vi "Monochromator.vi"() -> ()   [LabVIEW 2018]
uses:
  classes/Tushars Events Toolkit/Software/Modules/EventClient_ObjectReference.ctl
  Controls/Data highway.ctl
  Controls/LED intensity Command.ctl
  Strict Type Controls/Settings Operation.ctl
  Controls/API Command.ctl
  42e5cc38-9382-4005-a5db-d423bf5d2c61.vi
  dcdd8a02-0f9a-4db7-9287-66503d747d34.vi
  classes/Variable Manager/VariableManager_Bool.vi
  Controls/Support Global.vi
  classes/Variable Manager/VariableManager_I32.vi
  classes/Variable Manager/VariableManager_Double.vi
panel:
  out "Quit":bool
  out "error out":errorcluster
  in  "error in (no error)":errorcluster
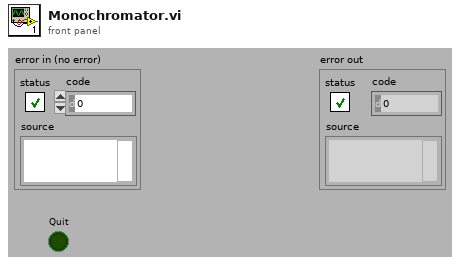
[diagram p1: front panel]
types:
  T1 = typedef "Data highway.ctl" = cluster{"MonoCr Port":refnum<visa-resource-name>, "Grating Selection":enum16{"Grating@1", "Grating@2"}, "Connection?":bool, "LED Comm":T2, "Intensity Value":i32, "Grating Number":i32, "Wavenumber":i32, "Slit Width":i32, "Filter Num":i32, "Grating Density":i32, "Wavelength(nm)":i32, "offset":dbl}
  T2 = typedef "LED intensity Command.ctl" = enum16{"LED@1", "LED@2"}
  T3 = typedef "EventClient_ObjectReference.ctl" = refnum<k1>
  T4 = typedef "API Command.ctl" = enum16{"Init", "Device Check", "Grating Density@1", "Grating Density@2", "SetWavelength", "Filter Selection", "Shutter open", "Shutter close", "LED Intensity", "Set Grating", "Slit Width", "Stop running", "Reset Mono", "Close"}
  T5 = typedef "Settings Operation.ctl" = enum8{"Get Value", "Set Value", "Read File", "Write File", "Write Stored Value"}
  T6 = typedef "Settings.ctl" = cluster{"Mono Cr":cluster{"Port":refnum<visa-resource-name>, "baud rate":u32, "data bits":u16, "parity":enum16{"None", "Odd", "Even", "Mark", "Space"}, "stop bits":u16, "flow control":u16, "timeout":u32}, "Merlin":cluster{"Port":refnum<visa-resource-name>, "baud rate":u32, "data bits":u16, "parity":enum16{"None", "Odd", "Even", "Mark", "Space"}, "stop bits":u16, "flow control":u16, "timeout":u32}}
  T7 = typedef "Wavelength Cluster Variable.ctl" = cluster{"Filter Num":i32, "Grating Density":i32, "Wavelength(nm)":i32}
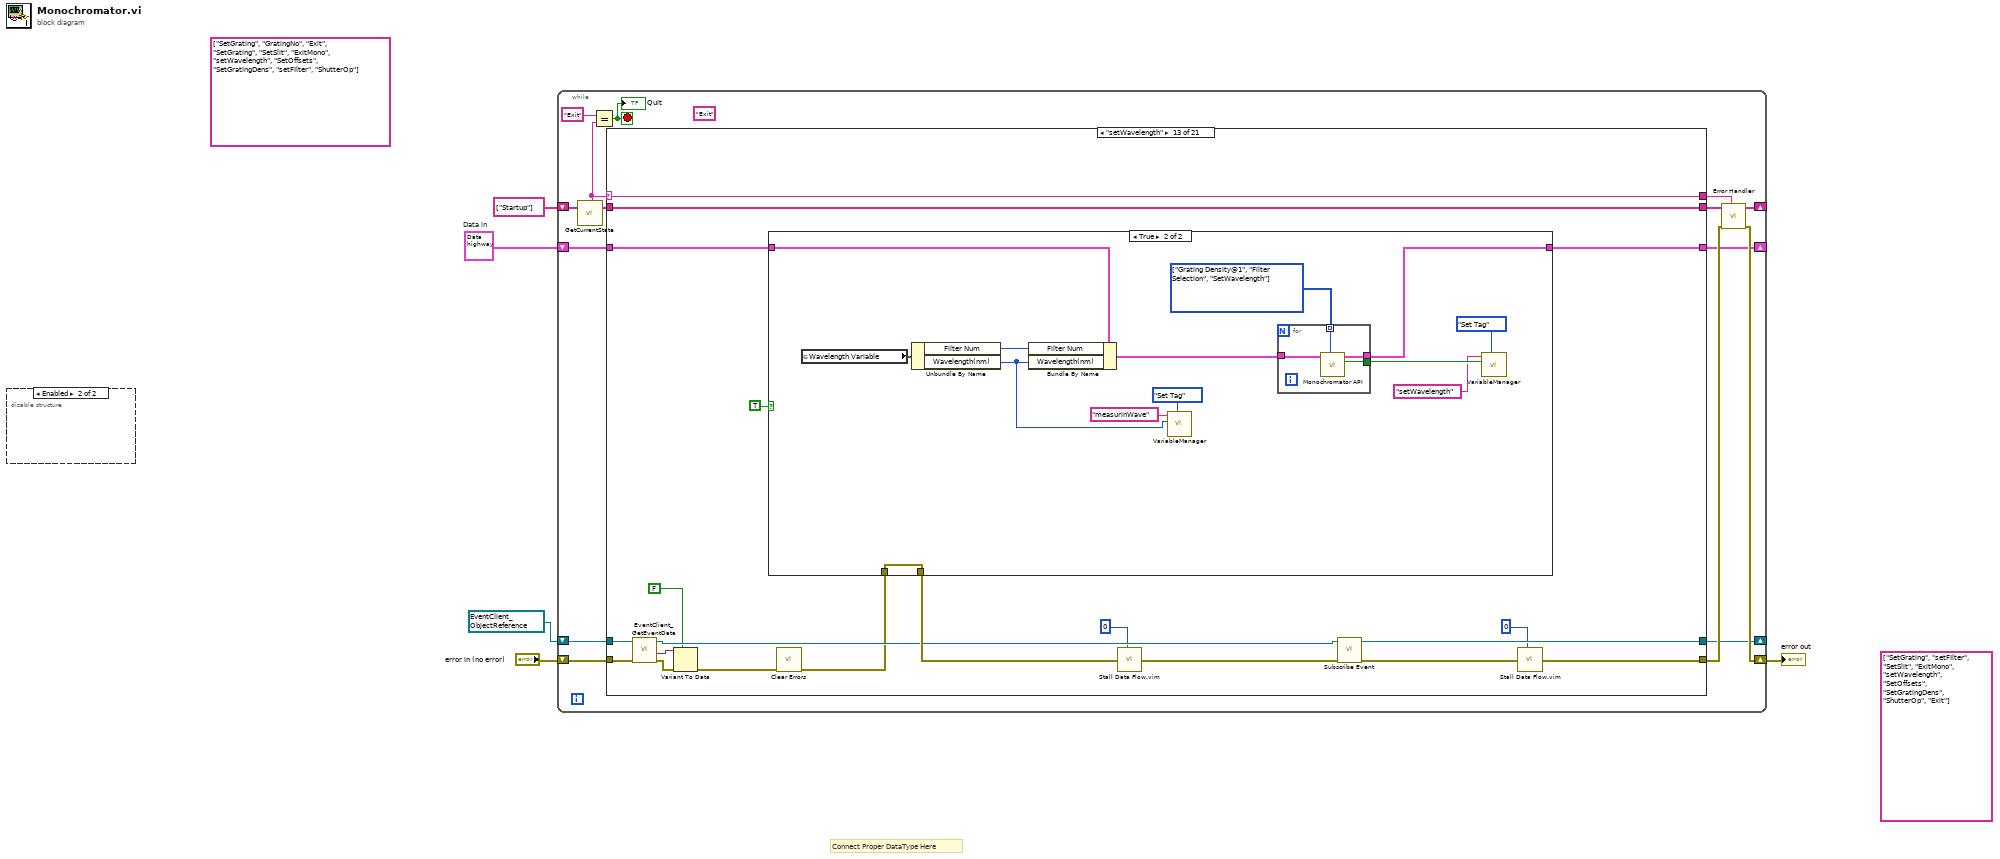
[diagram p0: block diagram]
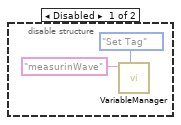
[diagram p2: hidden frame]
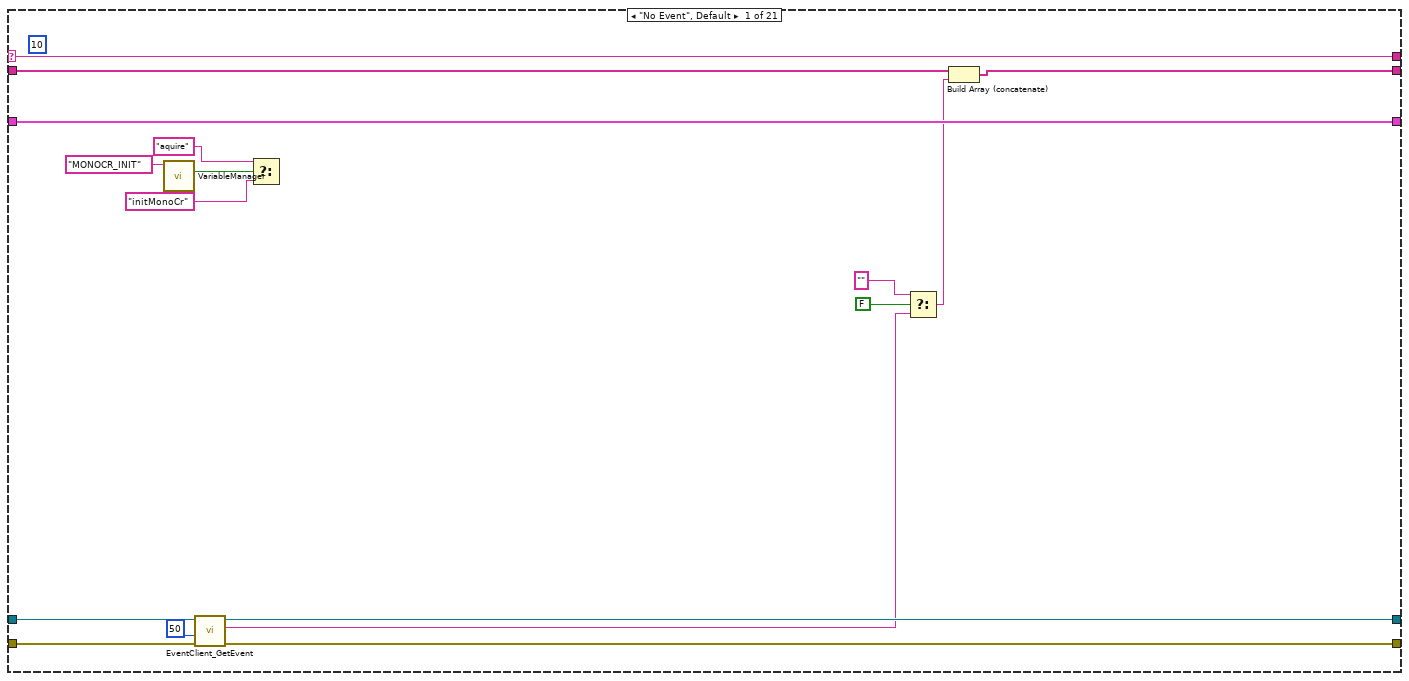
[diagram p3: hidden frame]
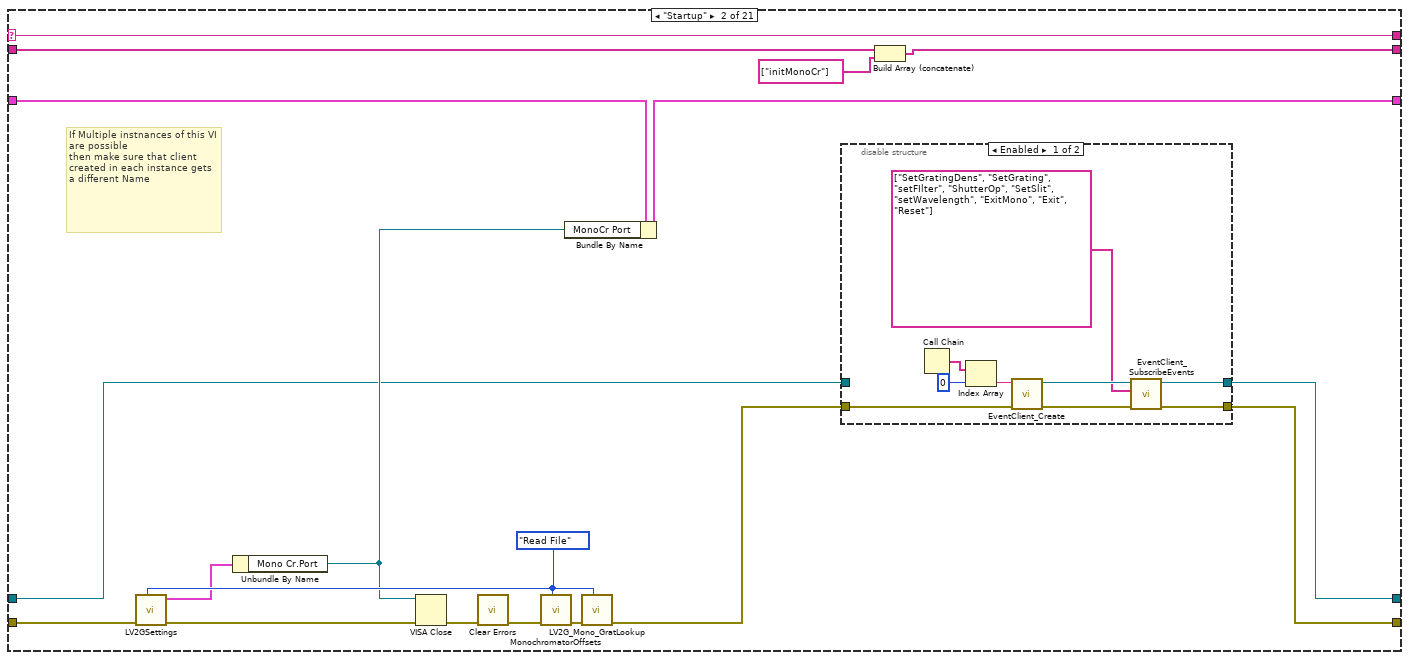
[diagram p4: hidden frame]
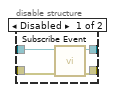
[diagram p6: hidden frame]
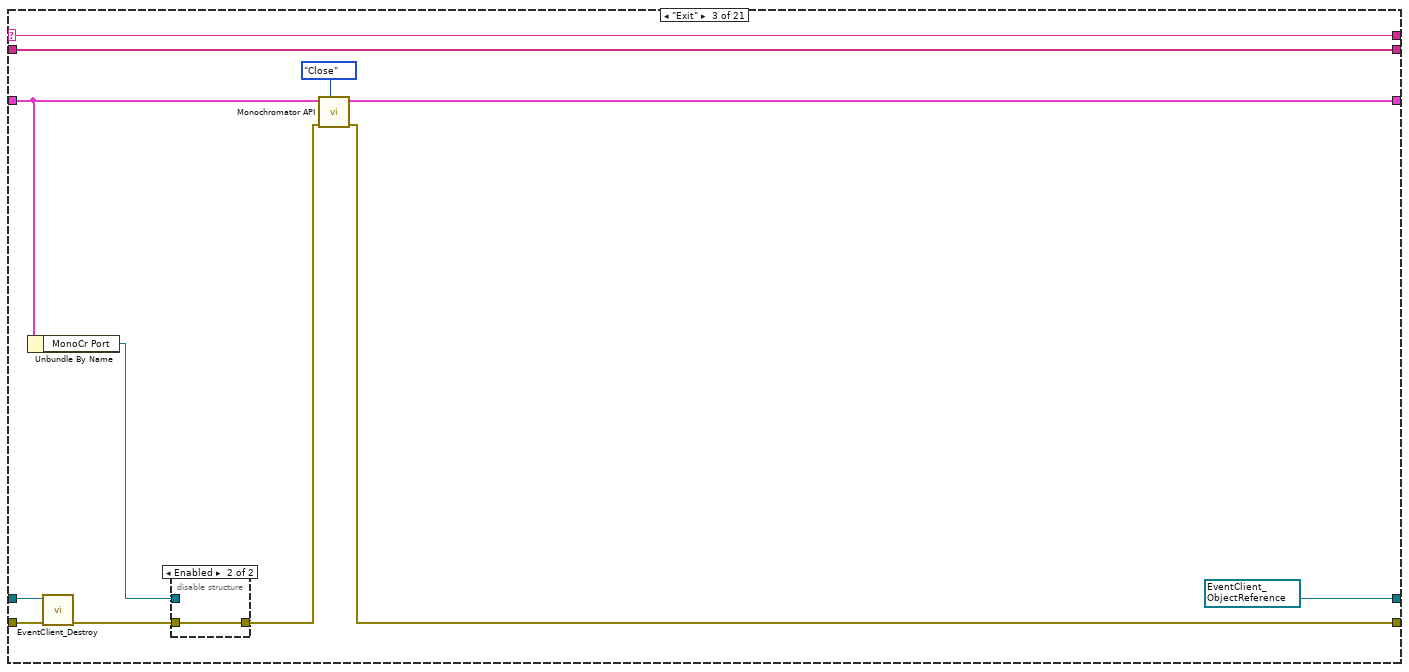
[diagram p7: hidden frame]
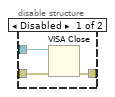
[diagram p8: hidden frame]
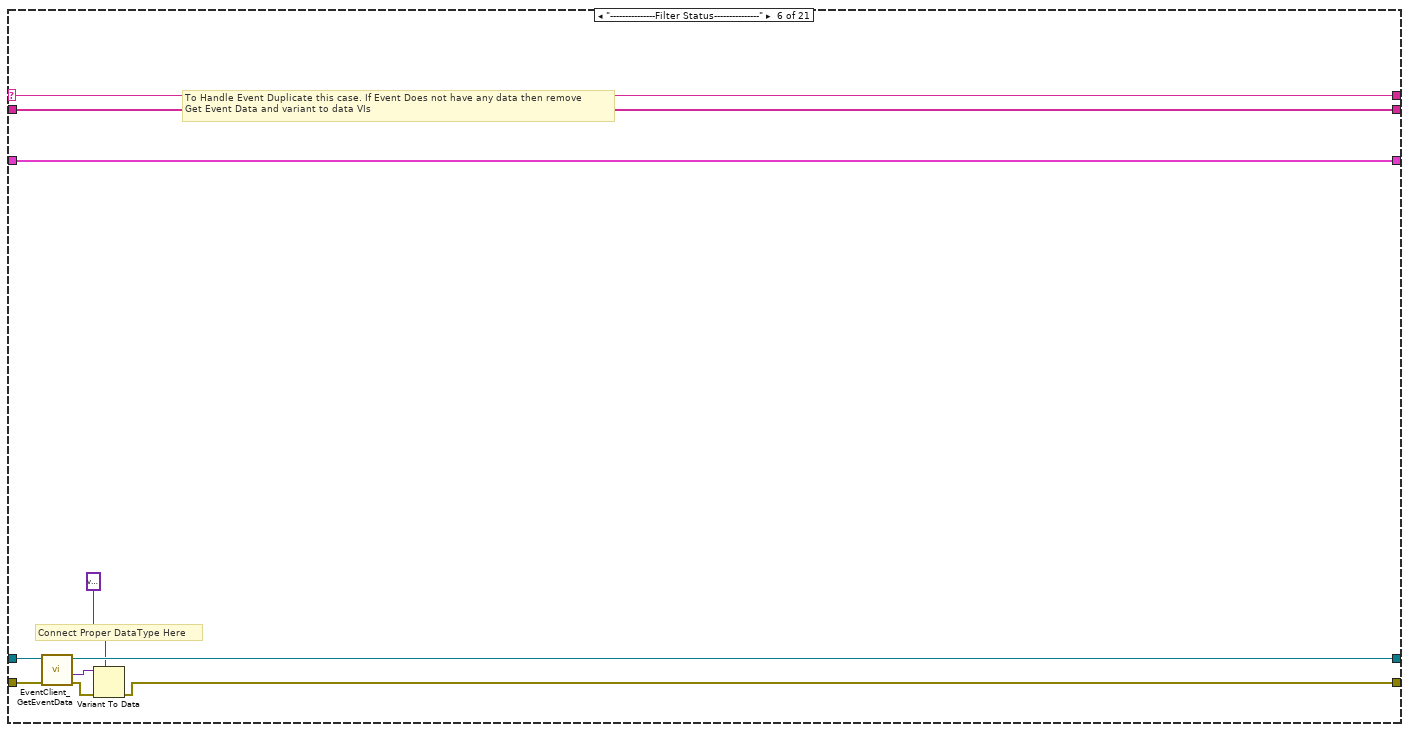
[diagram p11: hidden frame]
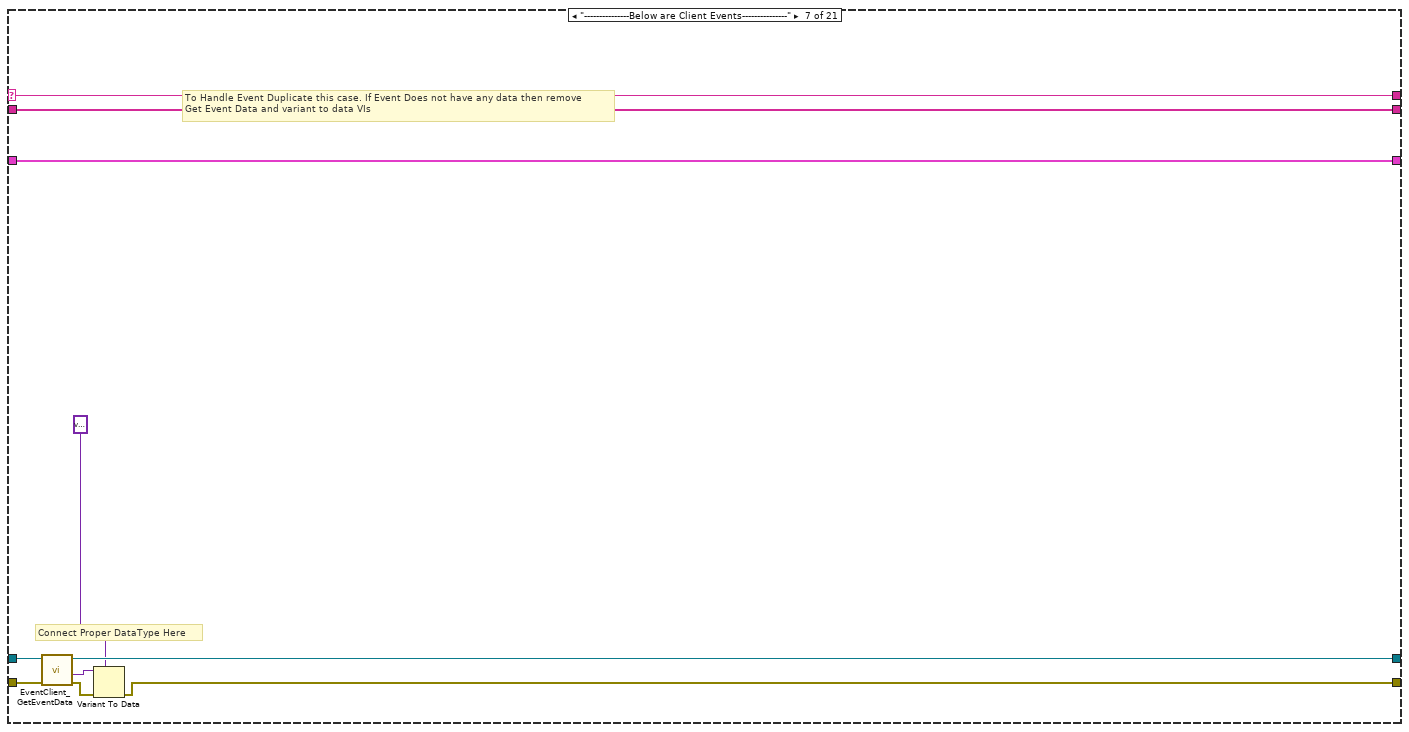
[diagram p12: hidden frame]
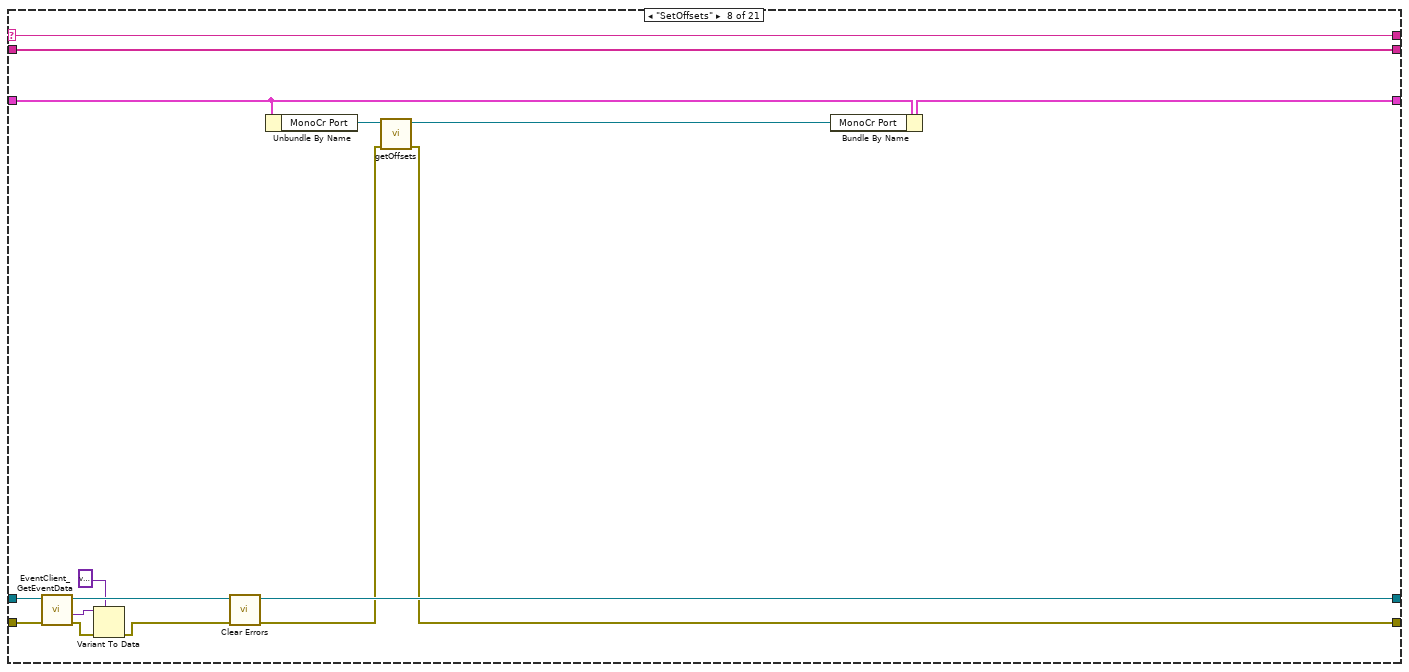
[diagram p13: hidden frame]
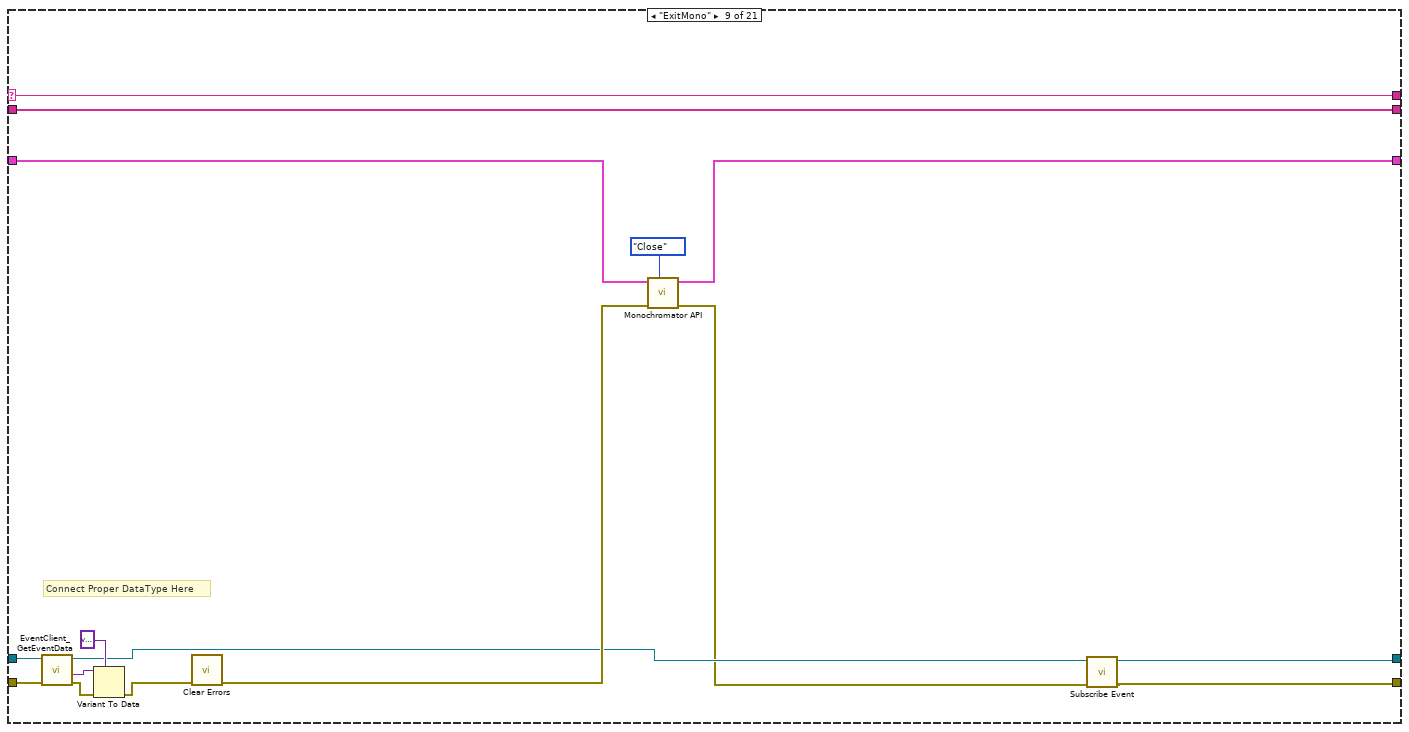
[diagram p14: hidden frame]
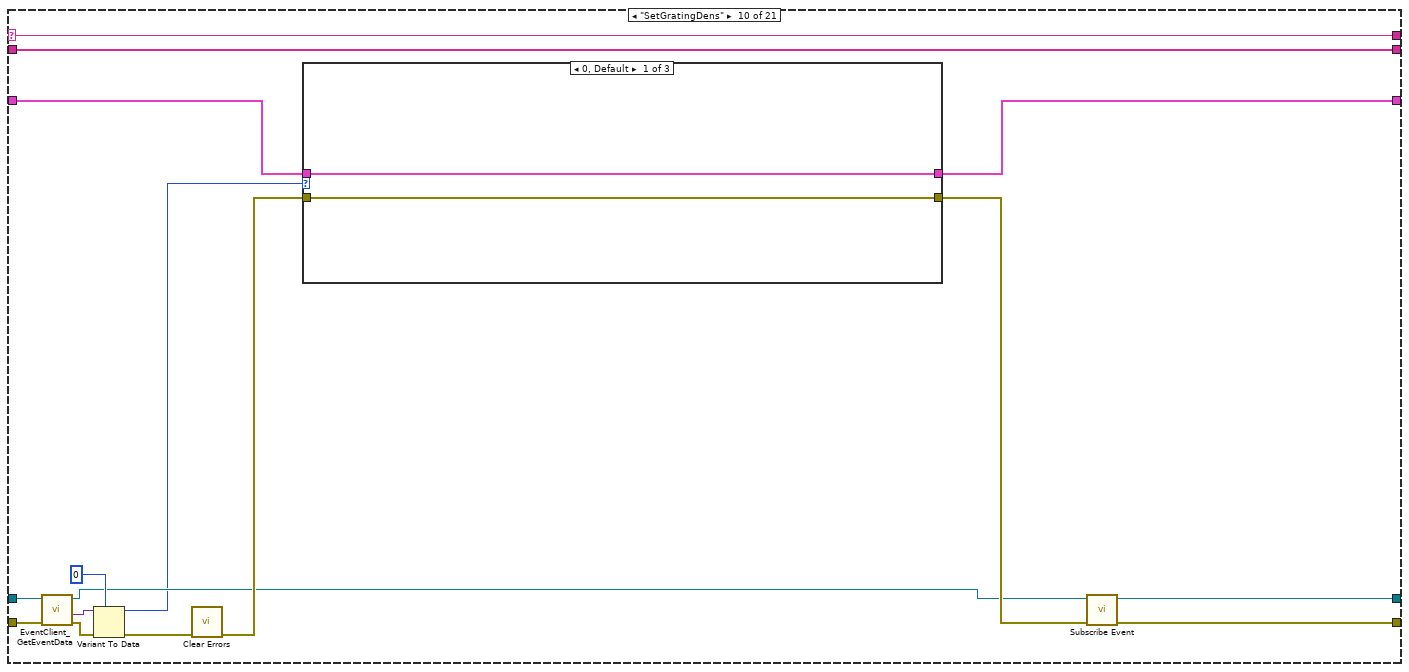
[diagram p15: hidden frame]
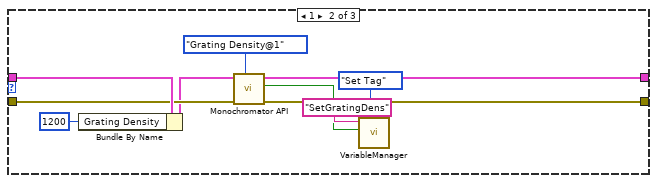
[diagram p16: hidden frame]
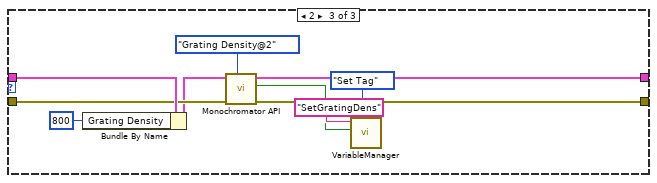
[diagram p17: hidden frame]
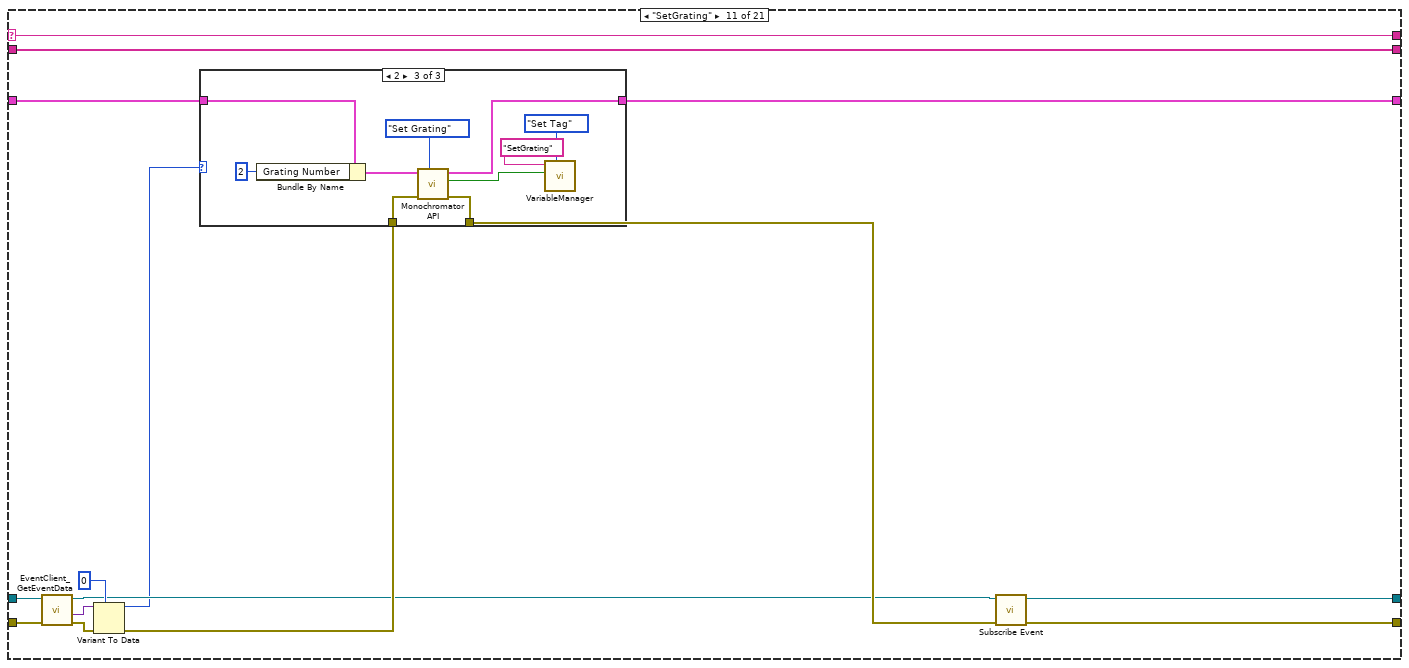
[diagram p18: hidden frame]
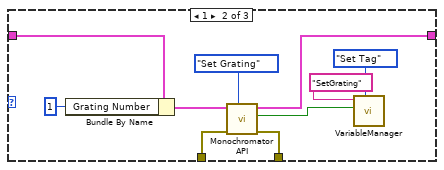
[diagram p20: hidden frame]
diagram:
  w1 = T1 {"MonoCr Port"="COM3", "Grating Selection"=enum."Grating@1", "Connection?"=TRUE, "LED Comm"=enum."LED@1", "Intensity Value"=20, "Grating Number"=1, "Wavenumber"=0, "Slit Width"=8, "Filter Num"=3, "Grating Density"=1200, "Wavelength(nm)"=532, "offset"=0.0}  # Data in
  (unwired) string[] ["SetGrating", "GratingNo", "Exit", "SetGrating", "SetSlit", "ExitMono", "setWavelength", "SetOffsets", "SetGratingDens", "setFIlter", "ShutterOp"] ("Events")
  (unwired) string[] ["SetGrating", "setFIlter", "SetSlit", "ExitMono", "setWavelength", "SetOffsets", "SetGratingDens", "ShutterOp", "Exit"] ("Events")
  w2 = T3 refnum items=["EventClient"] ("reference")
  # "Connect Proper DataType Here"
  n1 = disable-structure shown="Enabled" {
    frame Disabled {
      n2 = call-poly "VariableManager.vi"("Operation"=enum16{"Get Tag", "Set Tag"}."Set Tag", "Tag"="measurinWave") -> ()  [unwired: 5 in, 5 out]
    }
    frame Enabled {
    }
  }
  n3 = while {
    shift-right: [w18] -> _
    shift-left: string[] ["Startup"] ("State Array Out") -> [w22]
    shift-right: [w14] -> w3
    shift-left: "error in (no error)" -> [w15]
    shift-right: [w11] -> _
    shift-left: w2 -> [w10]
    shift-right: [w8] -> _
    shift-left: w1 -> [w9]
    stop <- w19 stop-if-true
    (unwired) "Exit" ("x")
    n4 = call "GetCurrentState.vi"("State Array In"=w22) -> ("Current State"=w12:string, "State Array Out"=w21:string[])  [unwired: 17 in]
    n5 = Equal?(x="Exit", y=w12) -> (x = y?=w19:bool)
    "Quit" <- w19
    n6 = case shown="\"setWavelength\"" w12 {
      selector: w12 -> [w39 w57 w88 w96 w101 w111 w121 w136 w152 w168 w205 w242 w344 w378 w450 w468 w483 w488 w507 w512 w530]
      tunnel: w21 -> [w31 w56 w87 w97 w102 w112 w122 w137 w153 w169 w206 w243 w345 w379 w451 w469 w484 w489 w502 w511 w517]
      tunnel: [w34 w55 w87 w97 w102 w112 w122 w137 w153 w169 w206 w243 w345 w379 w451 w469 w484 w489 w502 w511 w514] -> w17
      tunnel: [w36 w53 w78 w95 w100 w107 w117 w123 w139 w157 w195 w232 w329 w367 w435 w459 w482 w485 w501 w510 errorcluster {"status"=FALSE, "code"=0, "source"=""} ("error in (no error)")] -> w13
      tunnel: [w39 w57 w88 w96 w101 w111 w121 w136 w152 w168 w205 w242 w344 w378 w450 w468 w483 w488 w507 w512 w530] -> w16
      tunnel: w15 -> [w37 w50 w85 w95 w100 w109 w119 w134 w150 w166 w203 w240 w342 w376 w448 w466 w482 w485 w503 w510 w518]
      tunnel: [w35 w52 w84 w94 w99 w105 w115 w131 w138 w156 w194 w231 w334 w368 w434 w458 w481 w487 w506 w509 w516] -> w11
      tunnel: w10 -> [w38 w41 w86 w94 w99 w110 w120 w135 w151 w167 w204 w241 w343 w377 w449 w467 w481 w487 w506 w509 w516]
      tunnel: w9 -> [w32 w51 w80 w93 w98 w103 w113 w127 w144 w160 w200 w237 w339 w373 w445 w463 w480 w486 w500 w508 w515]
      tunnel: [w32 w46 w77 w93 w98 w103 w113 w126 w143 w162 w199 w236 w338 w372 w444 w462 w480 w486 w499 w508 w515] -> w8
      frame "No Event", Default {
        (unwired) 10
        n7 = call-poly "VariableManager.vi"("Tag"="MONOCR_INIT") -> ("Value out"=w28:bool)  [unwired: 7 in, 3 out]
        n8 = call "EventClient_GetEvent.vi"("error in (no error)"=w37, "timeout in ms (-1)"=50, "reference"=w38) -> ("error out"=w36:errorcluster, "Name"=w30:string, "reference out"=w35:T3)  [unwired: 4 in, 2 out]
        n9 = Select(t="aquire" ("Tag"), s=w28, f="initMonoCr" ("Tag")) -> ()  [unwired: 1 out]
        n10 = Select(t="", s=FALSE, f=w30) -> (s? t:f=w29:string)
        n11 = Build Array (concatenate)(w31, w29) -> (w34:string[])
      }
      frame "Startup" {
        w49 = Settings_Operation."Read File" ("Operation")
        # "If Multiple instnances of this VI are possible \nthen make sure that client created in each instance gets a different Name"
        n12 = call "LV2GSettings.vi"("Operation"=w49, "error in (no error)"=w50) -> ("error out"=w45:errorcluster, "Settings out"=w40:T6)  [unwired: 8 in]
        n13 = Unbundle By Name(w40) -> ("Mono Cr.Port"=w43:refnum<visa-resource-name>)
        n14 = VISA Close(VISA resource name=w43, error in (no error)=w45) -> (error out=w44:errorcluster)
        n15 = call <vilib>:"Clear Errors.vi"("error in (no error)"=w44) -> ("error out"=w42:errorcluster)  [unwired: 5 in, 1 out]
        n16 = call "MonochromatorOffsets.vi"("Operation"=w49, "error in (no error)"=w42) -> ("error out"=w48:errorcluster)  [unwired: 6 in, 3 out]
        n17 = Bundle By Name(cluster=w51, "MonoCr Port"=w43) -> (w46:T1)
        n18 = call "LV2G_Mono_GratLookup.vi"("Operation"=w49, "error in (no error)"=w48) -> ("error out"=w47:errorcluster)  [unwired: 7 in, 2 out]
        n19 = disable-structure shown="Enabled" {
          disable-tunnel: [w62 w68] -> w53
          disable-tunnel: [w60 w69] -> w52
          disable-tunnel: w47 -> [w59 w70]
          disable-tunnel: w41 -> [_ w67]
          frame Enabled {
            n20 = Call Chain() -> (call chain=w66:string[])
            n21 = Index Array(array=w66, index=0) -> (element=w64:string)
            n22 = call "EventClient_Create.vi"("error in (no error)"=w59, "Instance Name"=w64) -> ("error out"=w63:errorcluster, "reference"=w61:T3)  [unwired: 8 in]
            n23 = call "EventClient_SubscribeEvents.vi"("error in (no error)"=w63, "Events"=string[] ["SetGratingDens", "SetGrating", "setFIlter", "ShutterOp", "SetSlit", "setWavelength", "ExitMono", "Exit", "Reset"], "reference"=w61) -> ("error out"=w62:errorcluster, "reference out"=w60:T3)  [unwired: 7 in]
          }
          frame Disabled {
            n24 = disable-structure shown="Enabled" {
              disable-tunnel: w70 -> [w74 w75]
              disable-tunnel: [w73 w76] -> w69
              disable-tunnel: [w72 w75] -> w68
              disable-tunnel: w67 -> [w71 w76]
              frame Disabled {
                n25 = call "Subscribe Event.vi"("error in (no error)"=w74, "reference in"=w71) -> ("error out"=w72:errorcluster, "reference out"=w73:T3)  [unwired: 8 in]
              }
              frame Enabled {
              }
            }
          }
        }
        n26 = Build Array (concatenate)(w56, string[] ["initMonoCr"] ("State Array Out")) -> (w55:string[])
      }
      frame "Exit" {
        w84 = T3 refnum items=["EventClient"] ("reference out")
        n27 = Unbundle By Name(w80) -> ("MonoCr Port"=w82:refnum<visa-resource-name>)
        n28 = call "EventClient_Destroy.vi"("error in (no error)"=w85, "reference"=w86) -> ("error out"=w83:errorcluster)  [unwired: 9 in]
        n29 = disable-structure shown="Enabled" {
          disable-tunnel: w83 -> [w91 w92]
          disable-tunnel: w82 -> [w90 _]
          disable-tunnel: [w89 w92] -> w79
          frame Disabled {
            n30 = VISA Close(VISA resource name=w90, error in (no error)=w91) -> (error out=w89:errorcluster)
          }
          frame Enabled {
          }
        }
        n31 = call "Monochromator API.vi"("Comm"=API_Command."Close", "error in (no error)"=w79, "Data in out"=w80) -> ("error out"=w78:errorcluster, "Data in out"=w77:T1)  [unwired: 6 in, 1 out]
      }
      frame "---------------Below are UI Events---------------" {
        # "This State will never Execute\nIt is added just for improving code readability please do not remove this case"
      }
      frame "---------------Below are Menu Events---------------" {
        # "This State will never Execute\nIt is added just for improving code readability please do not remove this case"
      }
      frame "---------------Filter Status---------------" {
        # "To Handle Event Duplicate this case. If Event Does not have any data then remove\nGet Event Data and variant to data VIs"
        # "Connect Proper DataType Here"
        n32 = call "EventClient_GetEventData.vi"("error in (no error)"=w109, "reference"=w110) -> ("error out"=w108:errorcluster, "Data"=w106:variant, "reference out"=w105:T3)  [unwired: 7 in]
        n33 = Variant To Data(error in=w108, type=variant, Variant=w106) -> (error out=w107:errorcluster)  [unwired: 1 out]
      }
      frame "---------------Below are Client Events---------------" {
        # "To Handle Event Duplicate this case. If Event Does not have any data then remove\nGet Event Data and variant to data VIs"
        # "Connect Proper DataType Here"
        n34 = call "EventClient_GetEventData.vi"("error in (no error)"=w119, "reference"=w120) -> ("error out"=w118:errorcluster, "Data"=w116:variant, "reference out"=w115:T3)  [unwired: 7 in]
        n35 = Variant To Data(error in=w118, type=variant, Variant=w116) -> (error out=w117:errorcluster)  [unwired: 1 out]
      }
      frame "SetOffsets" {
        n36 = call "EventClient_GetEventData.vi"("error in (no error)"=w134, "reference"=w135) -> ("error out"=w133:errorcluster, "Data"=w132:variant, "reference out"=w131:T3)  [unwired: 7 in]
        n37 = Variant To Data(error in=w133, type=variant, Variant=w132) -> (error out=w125:errorcluster)  [unwired: 1 out]
        n38 = call <vilib>:"Clear Errors.vi"("error in (no error)"=w125) -> ("error out"=w124:errorcluster)  [unwired: 5 in, 1 out]
        n39 = Unbundle By Name(w127) -> ("MonoCr Port"=w129:refnum<visa-resource-name>)
        n40 = call "getOffsets.vi"("error in (no error)"=w124, "Port"=w129) -> ("error out"=w123:errorcluster, "Port out"=w128:refnum<visa-resource-name>)  [unwired: 8 in]
        n41 = Bundle By Name(cluster=w127, "MonoCr Port"=w128) -> (w126:T1)
      }
      frame "ExitMono" {
        # "Connect Proper DataType Here"
        n42 = call "EventClient_GetEventData.vi"("error in (no error)"=w150, "reference"=w151) -> ("error out"=w149:errorcluster, "Data"=w147:variant, "reference out"=w141:T3)  [unwired: 7 in]
        n43 = Variant To Data(error in=w149, type=variant, Variant=w147) -> (error out=w148:errorcluster)  [unwired: 1 out]
        n44 = call <vilib>:"Clear Errors.vi"("error in (no error)"=w148) -> ("error out"=w145:errorcluster)  [unwired: 5 in, 1 out]
        n45 = call "Monochromator API.vi"("Comm"=API_Command."Close", "error in (no error)"=w145, "Data in out"=w144) -> ("error out"=w140:errorcluster, "Data in out"=w143:T1)  [unwired: 6 in, 1 out]
        n46 = call "Subscribe Event.vi"("error in (no error)"=w140, "reference in"=w141) -> ("error out"=w139:errorcluster, "reference out"=w138:T3)  [unwired: 8 in]
      }
      frame "SetGratingDens" {
        n47 = call "EventClient_GetEventData.vi"("error in (no error)"=w166, "reference"=w167) -> ("error out"=w165:errorcluster, "Data"=w163:variant, "reference out"=w155:T3)  [unwired: 7 in]
        n48 = Variant To Data(error in=w165, type=0, Variant=w163) -> (data=w154:i32, error out=w164:errorcluster)
        n49 = call <vilib>:"Clear Errors.vi"("error in (no error)"=w164) -> ("error out"=w159:errorcluster)  [unwired: 5 in, 1 out]
        n50 = case shown="0, Default" w154 {
          tunnel: [w171 w181 w191] -> w162
          tunnel: w160 -> [w171 w176 w186]
          tunnel: w159 -> [w170 w175 w185]
          tunnel: [w170 w174 w184] -> w158
          frame 0, Default {
          }
          frame 1 {
            n51 = Bundle By Name(cluster=w176, "Grating Density"=1200) -> (w173:T1)
            n52 = call "Monochromator API.vi"("Comm"=API_Command."Grating Density@1", "error in (no error)"=w175, "Data in out"=w173) -> ("error out"=w174:errorcluster, "Connection?"=w178:bool, "Data in out"=w181:T1)  [unwired: 6 in]
            n53 = call-poly "VariableManager.vi"("Operation"=enum16{"Get Tag", "Set Tag"}."Set Tag", "Value"=w178, "Tag"="SetGratingDens" ("String")) -> ()  [unwired: 5 in, 4 out]
          }
          frame 2 {
            n54 = Bundle By Name(cluster=w186, "Grating Density"=800) -> (w183:T1)
            n55 = call "Monochromator API.vi"("Comm"=API_Command."Grating Density@2", "error in (no error)"=w185, "Data in out"=w183) -> ("error out"=w184:errorcluster, "Connection?"=w188:bool, "Data in out"=w191:T1)  [unwired: 6 in]
            n56 = call-poly "VariableManager.vi"("Operation"=enum16{"Get Tag", "Set Tag"}."Set Tag", "Value"=w188, "Tag"="SetGratingDens" ("String")) -> ()  [unwired: 5 in, 4 out]
          }
        }
        n57 = call "Subscribe Event.vi"("error in (no error)"=w158, "reference in"=w155) -> ("error out"=w157:errorcluster, "reference out"=w156:T3)  [unwired: 8 in]
      }
      frame "SetGrating" {
        n58 = call "EventClient_GetEventData.vi"("error in (no error)"=w203, "reference"=w204) -> ("error out"=w202:errorcluster, "Data"=w201:variant, "reference out"=w193:T3)  [unwired: 7 in]
        n59 = Variant To Data(error in=w202, type=0 ("GratingNo"), Variant=w201) -> (data=w192:i32, error out=w198:errorcluster)
        n60 = case shown="2" w192 {
          tunnel: w200 -> [w208 w218 w228]
          tunnel: [w208 w217 w227] -> w199
          tunnel: w198 -> [w207 w216 w226]
          tunnel: [w207 w210 w220] -> w196
          frame 0, Default {
          }
          frame 1 {
            n61 = Bundle By Name(cluster=w218, "Grating Number"=1) -> (w214:T1)
            n62 = call "Monochromator API.vi"("Comm"=API_Command."Set Grating", "error in (no error)"=w216, "Data in out"=w214) -> ("error out"=w210:errorcluster, "Connection?"=w211:bool, "Data in out"=w217:T1)  [unwired: 6 in]
            n63 = call-poly "VariableManager.vi"("Operation"=enum16{"Get Tag", "Set Tag"}."Set Tag", "Value"=w211, "Tag"="SetGrating" ("String")) -> ()  [unwired: 5 in, 4 out]
          }
          frame 2 {
            n64 = Bundle By Name(cluster=w228, "Grating Number"=2) -> (w224:T1)
            n65 = call "Monochromator API.vi"("Comm"=API_Command."Set Grating", "error in (no error)"=w226, "Data in out"=w224) -> ("error out"=w220:errorcluster, "Connection?"=w221:bool, "Data in out"=w227:T1)  [unwired: 6 in]
            n66 = call-poly "VariableManager.vi"("Operation"=enum16{"Get Tag", "Set Tag"}."Set Tag", "Value"=w221, "Tag"="SetGrating" ("String")) -> ()  [unwired: 5 in, 4 out]
          }
        }
        n67 = call "Subscribe Event.vi"("error in (no error)"=w196, "reference in"=w193) -> ("error out"=w195:errorcluster, "reference out"=w194:T3)  [unwired: 8 in]
      }
      frame "SetSlit" {
        n68 = call "EventClient_GetEventData.vi"("error in (no error)"=w240, "reference"=w241) -> ("error out"=w239:errorcluster, "Data"=w238:variant, "reference out"=w230:T3)  [unwired: 7 in]
        n69 = Variant To Data(error in=w239, type=0, Variant=w238) -> (data=w229:i32, error out=w235:errorcluster)
        n70 = case shown="8" w229 {
          tunnel: w237 -> [w245 w255 w265 w275 w285 w295 w305 w315 w325]
          tunnel: [w245 w254 w264 w274 w284 w294 w304 w314 w324] -> w236
          tunnel: w235 -> [w244 w253 w263 w273 w283 w293 w303 w313 w323]
          tunnel: [w244 w247 w257 w267 w277 w287 w297 w307 w317] -> w233
          frame 0, Default {
          }
          frame 1 {
            n71 = Bundle By Name(cluster=w255, "Slit Width"=1) -> (w251:T1)
            n72 = call "Monochromator API.vi"("Comm"=API_Command."Slit Width", "error in (no error)"=w253, "Data in out"=w251) -> ("error out"=w247:errorcluster, "Connection?"=w248:bool, "Data in out"=w254:T1)  [unwired: 6 in]
            n73 = call-poly "VariableManager.vi"("Operation"=enum16{"Get Tag", "Set Tag"}."Set Tag", "Value"=w248, "Tag"="SetSlit" ("String")) -> ()  [unwired: 5 in, 4 out]
          }
          frame 2 {
            n74 = Bundle By Name(cluster=w265, "Slit Width"=2) -> (w261:T1)
            n75 = call "Monochromator API.vi"("Comm"=API_Command."Slit Width", "error in (no error)"=w263, "Data in out"=w261) -> ("error out"=w257:errorcluster, "Connection?"=w258:bool, "Data in out"=w264:T1)  [unwired: 6 in]
            n76 = call-poly "VariableManager.vi"("Operation"=enum16{"Get Tag", "Set Tag"}."Set Tag", "Value"=w258, "Tag"="SetSlit" ("String")) -> ()  [unwired: 5 in, 4 out]
          }
          frame 3 {
            n77 = Bundle By Name(cluster=w275, "Slit Width"=3) -> (w271:T1)
            n78 = call "Monochromator API.vi"("Comm"=API_Command."Slit Width", "error in (no error)"=w273, "Data in out"=w271) -> ("error out"=w267:errorcluster, "Connection?"=w268:bool, "Data in out"=w274:T1)  [unwired: 6 in]
            n79 = call-poly "VariableManager.vi"("Operation"=enum16{"Get Tag", "Set Tag"}."Set Tag", "Value"=w268, "Tag"="SetSlit" ("String")) -> ()  [unwired: 5 in, 4 out]
          }
          frame 4 {
            n80 = Bundle By Name(cluster=w285, "Slit Width"=4) -> (w281:T1)
            n81 = call "Monochromator API.vi"("Comm"=API_Command."Slit Width", "error in (no error)"=w283, "Data in out"=w281) -> ("error out"=w277:errorcluster, "Connection?"=w278:bool, "Data in out"=w284:T1)  [unwired: 6 in]
            n82 = call-poly "VariableManager.vi"("Operation"=enum16{"Get Tag", "Set Tag"}."Set Tag", "Value"=w278, "Tag"="SetSlit" ("String")) -> ()  [unwired: 5 in, 4 out]
          }
          frame 5 {
            n83 = Bundle By Name(cluster=w295, "Slit Width"=5) -> (w291:T1)
            n84 = call "Monochromator API.vi"("Comm"=API_Command."Slit Width", "error in (no error)"=w293, "Data in out"=w291) -> ("error out"=w287:errorcluster, "Connection?"=w288:bool, "Data in out"=w294:T1)  [unwired: 6 in]
            n85 = call-poly "VariableManager.vi"("Operation"=enum16{"Get Tag", "Set Tag"}."Set Tag", "Value"=w288, "Tag"="SetSlit" ("String")) -> ()  [unwired: 5 in, 4 out]
          }
          frame 6 {
            n86 = Bundle By Name(cluster=w305, "Slit Width"=6) -> (w301:T1)
            n87 = call "Monochromator API.vi"("Comm"=API_Command."Slit Width", "error in (no error)"=w303, "Data in out"=w301) -> ("error out"=w297:errorcluster, "Connection?"=w298:bool, "Data in out"=w304:T1)  [unwired: 6 in]
            n88 = call-poly "VariableManager.vi"("Operation"=enum16{"Get Tag", "Set Tag"}."Set Tag", "Value"=w298, "Tag"="SetSlit" ("String")) -> ()  [unwired: 5 in, 4 out]
          }
          frame 7 {
            n89 = Bundle By Name(cluster=w315, "Slit Width"=7) -> (w311:T1)
            n90 = call "Monochromator API.vi"("Comm"=API_Command."Slit Width", "error in (no error)"=w313, "Data in out"=w311) -> ("error out"=w307:errorcluster, "Connection?"=w308:bool, "Data in out"=w314:T1)  [unwired: 6 in]
            n91 = call-poly "VariableManager.vi"("Operation"=enum16{"Get Tag", "Set Tag"}."Set Tag", "Value"=w308, "Tag"="SetSlit" ("String")) -> ()  [unwired: 5 in, 4 out]
          }
          frame 8 {
            n92 = Bundle By Name(cluster=w325, "Slit Width"=8) -> (w321:T1)
            n93 = call "Monochromator API.vi"("Comm"=API_Command."Slit Width", "error in (no error)"=w323, "Data in out"=w321) -> ("error out"=w317:errorcluster, "Connection?"=w318:bool, "Data in out"=w324:T1)  [unwired: 6 in]
            n94 = call-poly "VariableManager.vi"("Operation"=enum16{"Get Tag", "Set Tag"}."Set Tag", "Value"=w318, "Tag"="SetSlit" ("String")) -> ()  [unwired: 5 in, 4 out]
          }
        }
        n95 = call "Subscribe Event.vi"("error in (no error)"=w233, "reference in"=w230) -> ("error out"=w232:errorcluster, "reference out"=w231:T3)  [unwired: 8 in]
      }
      frame "setWavelength" {
        n96 = call "EventClient_GetEventData.vi"("error in (no error)"=w342, "reference"=w343) -> ("error out"=w341:errorcluster, "Data"=w340:variant, "reference out"=w333:T3)  [unwired: 7 in]
        n97 = Variant To Data(error in=w341, type=FALSE, Variant=w340) -> (error out=w337:errorcluster)  [unwired: 1 out]
        n98 = call <vilib>:"Clear Errors.vi"("error in (no error)"=w337) -> ("error out"=w332:errorcluster)  [unwired: 5 in, 1 out]
        n99 = case shown="True" TRUE {
          tunnel: w339 -> [w347 w360]
          tunnel: [w347 w352] -> w338
          tunnel: w332 -> [w346 w351]
          tunnel: [w346 w351] -> w336
          frame False {
          }
          frame True {
            w354 = T4[] [enum."Grating Density@1", enum."Filter Selection", enum."SetWavelength"] items=["Init", "Device Check", "Grating Density@1", "Grating Density@2", "SetWavelength", "Filter Selection", "Shutter open", "Shutter close", "LED Intensity", "Set Grating", "Slit Width", "Stop running", "Reset Mono", "Close"] ("Comm")
            n100 = global read "Support Global.vi" "Wavelength Variable"() -> (w350:T7)
            n101 = Unbundle By Name(w350) -> ("Filter Num"=w349:i32, "Wavelength(nm)"=w348:i32)
            n102 = Bundle By Name(cluster=w360, "Filter Num"=w349, "Wavelength(nm)"=w348) -> (w353:T1)
            n103 = call-poly "VariableManager.vi"("Operation"=enum16{"Get Tag", "Set Tag"}."Set Tag", "Value"=w348, "Tag"="measurinWave") -> ()  [unwired: 5 in, 4 out]
            n104 = for {
              tunnel: [w364] -> w358
              tunnel: w354 -> [w363] mode=indexing
              tunnel: w353 -> [w362]
              tunnel: [w361] -> w352
              n105 = call "Monochromator API.vi"("Comm"=w363, "Data in out"=w362) -> ("Connection?"=w364:bool, "Data in out"=w361:T1)  [unwired: 7 in, 1 out]
            }
            n106 = call-poly "VariableManager.vi"("Operation"=enum16{"Get Tag", "Set Tag"}."Set Tag", "Value"=w358, "Tag"="setWavelength" ("String")) -> ()  [unwired: 5 in, 4 out]
          }
        }
        n107 = call "Stall Data Flow.vim"("value in"=w336, "milliseconds to wait"=u32 0) -> ("value out"=w331:errorcluster)  [unwired: 1 out]
        n108 = call "Subscribe Event.vi"("error in (no error)"=w331, "reference in"=w333) -> ("error out"=w335:errorcluster, "reference out"=w334:T3)  [unwired: 8 in]
        n109 = call "Stall Data Flow.vim"("value in"=w335, "milliseconds to wait"=u32 0) -> ("value out"=w329:errorcluster)  [unwired: 1 out]
      }
      frame "setFIlter" {
        n110 = call "EventClient_GetEventData.vi"("error in (no error)"=w376, "reference"=w377) -> ("error out"=w375:errorcluster, "Data"=w374:variant, "reference out"=w366:T3)  [unwired: 7 in]
        n111 = Variant To Data(error in=w375, type=0 ("wavelength"), Variant=w374) -> (data=w365:i32, error out=w371:errorcluster)
        n112 = case shown="3" w365 {
          tunnel: w373 -> [w381 w391 w401 w411 w421 w431]
          tunnel: [w381 w390 w400 w410 w420 w430] -> w372
          tunnel: w371 -> [w380 w389 w399 w409 w419 w429]
          tunnel: [w380 w383 w393 w403 w413 w423] -> w369
          frame 0, Default {
          }
          frame 1 {
            n113 = Bundle By Name(cluster=w391, "Filter Num"=1) -> (w388:T1)
            n114 = call "Monochromator API.vi"("Comm"=API_Command."Filter Selection", "error in (no error)"=w389, "Data in out"=w388) -> ("error out"=w383:errorcluster, "Connection?"=w384:bool, "Data in out"=w390:T1)  [unwired: 6 in]
            n115 = call-poly "VariableManager.vi"("Operation"=enum16{"Get Tag", "Set Tag"}."Set Tag", "Value"=w384, "Tag"="setFIlter" ("String")) -> ()  [unwired: 5 in, 4 out]
          }
          frame 2 {
            n116 = Bundle By Name(cluster=w401, "Filter Num"=2) -> (w398:T1)
            n117 = call "Monochromator API.vi"("Comm"=API_Command."Filter Selection", "error in (no error)"=w399, "Data in out"=w398) -> ("error out"=w393:errorcluster, "Connection?"=w394:bool, "Data in out"=w400:T1)  [unwired: 6 in]
            n118 = call-poly "VariableManager.vi"("Operation"=enum16{"Get Tag", "Set Tag"}."Set Tag", "Value"=w394, "Tag"="setFIlter" ("String")) -> ()  [unwired: 5 in, 4 out]
          }
          frame 3 {
            n119 = Bundle By Name(cluster=w411, "Filter Num"=3) -> (w408:T1)
            n120 = call "Monochromator API.vi"("Comm"=API_Command."Filter Selection", "error in (no error)"=w409, "Data in out"=w408) -> ("error out"=w403:errorcluster, "Connection?"=w404:bool, "Data in out"=w410:T1)  [unwired: 6 in]
            n121 = call-poly "VariableManager.vi"("Operation"=enum16{"Get Tag", "Set Tag"}."Set Tag", "Value"=w404, "Tag"="setFIlter" ("String")) -> ()  [unwired: 5 in, 4 out]
          }
          frame 4 {
            n122 = Bundle By Name(cluster=w421, "Filter Num"=4) -> (w418:T1)
            n123 = call "Monochromator API.vi"("Comm"=API_Command."Filter Selection", "error in (no error)"=w419, "Data in out"=w418) -> ("error out"=w413:errorcluster, "Connection?"=w414:bool, "Data in out"=w420:T1)  [unwired: 6 in]
            n124 = call-poly "VariableManager.vi"("Operation"=enum16{"Get Tag", "Set Tag"}."Set Tag", "Value"=w414, "Tag"="setFIlter" ("String")) -> ()  [unwired: 5 in, 4 out]
          }
          frame 5 {
            n125 = Bundle By Name(cluster=w431, "Filter Num"=5) -> (w428:T1)
            n126 = call "Monochromator API.vi"("Comm"=API_Command."Filter Selection", "error in (no error)"=w429, "Data in out"=w428) -> ("error out"=w423:errorcluster, "Connection?"=w424:bool, "Data in out"=w430:T1)  [unwired: 6 in]
            n127 = call-poly "VariableManager.vi"("Operation"=enum16{"Get Tag", "Set Tag"}."Set Tag", "Value"=w424, "Tag"="setFIlter" ("String")) -> ()  [unwired: 5 in, 4 out]
          }
        }
        n128 = call "Subscribe Event.vi"("error in (no error)"=w369, "reference in"=w366) -> ("error out"=w367:errorcluster, "reference out"=w368:T3)  [unwired: 8 in]
      }
      frame "ShutterOp" {
        n129 = call "EventClient_GetEventData.vi"("error in (no error)"=w448, "reference"=w449) -> ("error out"=w447:errorcluster, "Data"=w446:variant, "reference out"=w433:T3)  [unwired: 7 in]
        n130 = Variant To Data(error in=w447, type=enum16{"Open", "Close"}."Open" ("Shutter"), Variant=w446) -> (data=w441:enum16{"Open", "Close"}, error out=w443:errorcluster)
        n131 = call <vilib>:"Clear Errors.vi"("error in (no error)"=w443) -> ("error out"=w432:errorcluster)  [unwired: 5 in, 1 out]
        n132 = case shown="\"Open\", Default" w441 {
          tunnel: [API_Command."Shutter open" ("Comm") API_Command."Shutter close" ("Comm")] -> w440
          frame "Open", Default {
          }
          frame "Close" {
          }
        }
        n133 = call "Monochromator API.vi"("Comm"=w440, "error in (no error)"=w432, "Data in out"=w445) -> ("error out"=w436:errorcluster, "Connection?"=w437:bool, "Data in out"=w444:T1)  [unwired: 6 in]
        n134 = call-poly "VariableManager.vi"("Operation"=enum16{"Get Tag", "Set Tag"}."Set Tag", "Value"=w437, "Tag"="ShutterOp" ("String")) -> ()  [unwired: 5 in, 4 out]
        n135 = call "Subscribe Event.vi"("error in (no error)"=w436, "reference in"=w433) -> ("error out"=w435:errorcluster, "reference out"=w434:T3)  [unwired: 8 in]
      }
      frame "Reset" {
        n136 = call "EventClient_GetEventData.vi"("error in (no error)"=w466, "reference"=w467) -> ("error out"=w465:errorcluster, "Data"=w464:variant, "reference out"=w457:T3)  [unwired: 7 in]
        n137 = Variant To Data(error in=w465, type=FALSE, Variant=w464) -> (data=w454:bool, error out=w461:errorcluster)
        n138 = call <vilib>:"Clear Errors.vi"("error in (no error)"=w461) -> ("error out"=w456:errorcluster)  [unwired: 5 in, 1 out]
        n139 = case shown="True" w454 {
          tunnel: w463 -> [w470 w479]
          tunnel: [w470 w478] -> w462
          tunnel: [w471 w474] -> w460
          tunnel: w456 -> [w471 w473]
          frame False {
          }
          frame True {
            n140 = call "Monochromator API.vi"("Comm"=API_Command."Reset Mono", "error in (no error)"=w473, "Data in out"=w479) -> ("error out"=w474:errorcluster, "Connection?"=w475:bool, "Data in out"=w478:T1)  [unwired: 6 in]
            n141 = call-poly "VariableManager.vi"("Operation"=enum16{"Get Tag", "Set Tag"}."Set Tag", "Value"=w475, "Tag"="Reset" ("String")) -> ()  [unwired: 5 in, 4 out]
          }
        }
        n142 = call "Subscribe Event.vi"("error in (no error)"=w460, "reference in"=w457) -> ("error out"=w459:errorcluster, "reference out"=w458:T3)  [unwired: 8 in]
      }
      frame "---------------Below are Subroutine states---------------" {
      }
      frame "aquire" {
        n143 = disable-structure shown="Disabled" {
          disable-tunnel: w485 -> [w491 _]
          frame Disabled {
            n144 = Unbundle(w491) -> ("status"=w493:bool)  [unwired: 2 out]
            n145 = Not(x=w493) -> (.not. x?=w494:bool)
            n146 = call-poly "VariableManager.vi"("Operation"=enum16{"Get Tag", "Set Tag"}."Set Tag", "Value"=w494, "Tag"="MONOCR_INIT") -> ()  [unwired: 5 in, 4 out]
          }
          frame Enabled {
          }
        }
      }
      frame "initMonoCr" {
        n147 = Unbundle By Name(w500) -> ("MonoCr Port"=w504:refnum<visa-resource-name>)
        n148 = VISA Close(VISA resource name=w504) -> (error out=w505:errorcluster)  [unwired: 1 in]
        n149 = call <vilib>:"Clear Errors.vi"("error in (no error)"=w505) -> ()  [unwired: 5 in, 2 out]
        n150 = call "Monochromator API.vi"("Comm"=API_Command."Device Check", "error in (no error)"=w503, "Data in out"=w500) -> ("error out"=w501:errorcluster, "Connection?"=w496:bool, "Data in out"=w499:T1)  [unwired: 6 in]
        n151 = call-poly "VariableManager.vi"("Operation"=enum16{"Get Tag", "Set Tag"}."Set Tag", "Value"=w496, "Tag"="MONOCR_INIT") -> ()  [unwired: 5 in, 4 out]
      }
      frame "---------------Below are Error Handling VIs---------------" {
      }
      frame "Error" {
        n152 = Call Chain() -> (call chain=w525:string[])
        n153 = for {
          tunnel: w525 -> [w533] mode=indexing
          shift-right: [w531] -> w522
          shift-left: "" -> [w534]
          n154 = Concatenate Strings(w534, w533, " -> ") -> (w531:string)
        }
        n155 = Unbundle By Name(w518) -> ("code"=w520:i32, "source"=w519:string)
        n156 = Match Pattern(string=w519, regular expression=":") -> (before substring=w523:string, after substring=w527:string)  [unwired: 1 in, 2 out]
        n157 = Build Array (concatenate)(w517, "Exit" ("x")) -> (w514:string[])
        n158 = Format Into String(format string="Error Occured In\"%s\" state of \"%s\" VI\nError Code: %d\nError Description: \"%s\"", w523, w522, w520, w527) -> (resulting string=w526:string)  [unwired: 2 in, 1 out]
        n159 = One Button Dialog(message=w526) -> ()  [unwired: 1 in, 1 out]
      }
    }
    n160 = call "Error Handler.vi"("Current State"=w16, "error in (no error)"=w13, "Msg Queue In"=w17) -> ("error out"=w14:errorcluster, "Msg Queue Out"=w18:string[])  [unwired: 7 in]
  }
  "error out" <- w3
